vi "Exponential Window.vi"   [LabVIEW 2020, in "NI_AALPro.lvlib"]
doc: "Applies an exponential window to the input signal <B>X</B>. Wire data to the <B>X</B> input to determine the polymorphic instance to use or manually select the instance."
uses:
  <vilib>/Analysis/NI_AALPro.lvlib
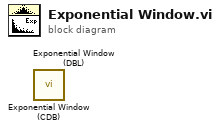
[diagram p0: block diagram]
diagram:
  n1 = call <vilib>:"Exponential Window (CDB).vi"() -> ()  [unwired: 2 in, 2 out]
  n2 = call <vilib>:"Exponential Window (DBL).vi"() -> ()  [unwired: 2 in, 2 out]
